vi "ParseIt.vi"(10 "Header Info":T1={"TFRFHeader"={"index"=22, "Xr"=294.1319931548027, "Yr"=349.0, "XActual"=294.1319931548027, "YActual"=349.0}, "Frequency Axis"={"Hz Resolution"=0.67291259765625, "Start Freq"=24.89776611328125, "End Freq"=3500.4913330078125}, "TSingleArray"={"fComplex"=1, "fLength"=5166.0, "a[2]"=0.0, "fConditionCheck"=1.0, "Precision"=0.0, "MtxVecVersion"=420.0, "SizeOf(TSample)"=8.0, "Tag"=0.0, "MtxVecFileCode"=64019.0, "a[9]"=0.0, "a[10]"=0.0}, "caption"="\u0000\u0000\u0000\u0000"}, 11 "Array":dbl[](array[numeric])) -> (1 "Waveform Graph":T2(graph), 2 "coherence":T2(graph), 3 "output array":dbl[][](array[numeric]), 4 "Complex FRF":cluster{"t0":dbl, "dt":dbl, "Y":cdb[]}, 5 "Number of bytes":dbl, 6 "run":cluster{"Sampling rate":dbl, "npts":dbl})   [LabVIEW 2022 SP3]
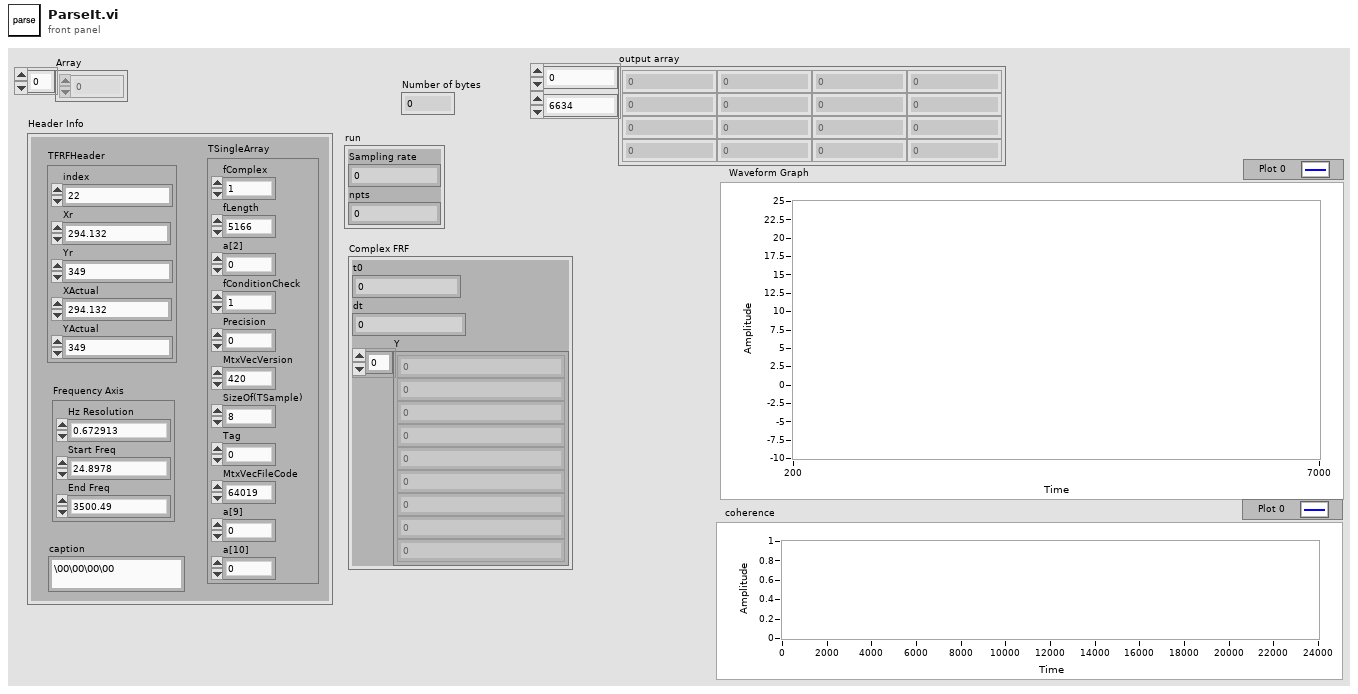
[diagram p1: front panel]
types:
  T1 = cluster{"TFRFHeader":cluster{"index":u32, "Xr":dbl, "Yr":dbl, "XActual":dbl, "YActual":dbl}, "Frequency Axis":cluster{"Hz Resolution":dbl, "Start Freq":dbl, "End Freq":dbl}, "TSingleArray":cluster{"fComplex":u32, "fLength":dbl, "a[2]":dbl, "fConditionCheck":dbl, "Precision":dbl, "MtxVecVersion":dbl, "SizeOf(TSample)":dbl, "Tag":dbl, "MtxVecFileCode":dbl, "a[9]":dbl, "a[10]":dbl}, "caption":string}
  T2 = cluster{"Start freq":dbl, "Hz resolution":dbl, dbl[]}
  T3 = cluster{"Start Freq":dbl, "Hz Resolution":dbl, cdb[]}
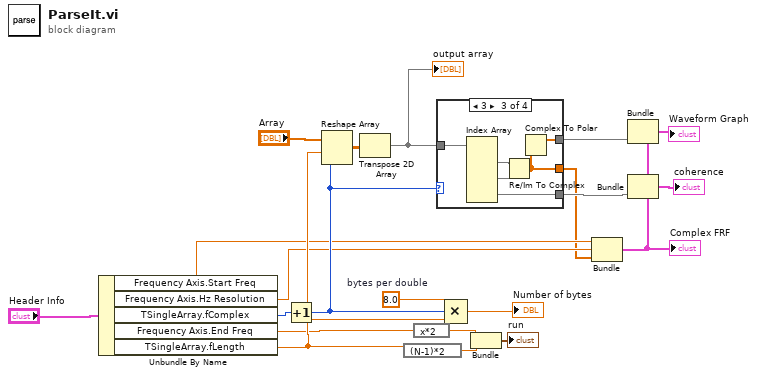
[diagram p0: block diagram]
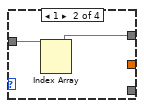
[diagram p3: hidden frame]
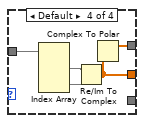
[diagram p4: hidden frame]
diagram:
  w11 = 8.0  # bytes per double
  n1 = Unbundle By Name("Header Info") -> ("Frequency Axis.Start Freq"=w3:dbl, "Frequency Axis.Hz Resolution"=w4:dbl, "TSingleArray.fComplex"=w16:u32, "Frequency Axis.End Freq"=w9:dbl, "TSingleArray.fLength"=w17:dbl)
  n2 = Increment(x=w16) -> (x+1=w19:u32)
  n3 = Reshape Array("Array", w17, w19) -> (w18:dbl[][])
  n4 = Transpose 2D Array(2D array=w18) -> (transposed array=w20:dbl[][])
  "output array" <- w20
  n5 = expression code="(N-1)*2"(w17) -> (w10:dbl)
  n6 = expression code="x*2"(w9) -> (w7:dbl)
  n7 = case shown="3" w19 {
    tunnel: w20 -> [_ w23 w29 w34]
    tunnel: [_ w22 w26 w31] -> w1
    tunnel: [_ _ w25 _] -> w21
    tunnel: [_ _ w24 w30] -> w2
    frame 0 {
    }
    frame 1 {
      n8 = Index Array(array=w23) -> (element=w22:dbl[])  [unwired: 2 in]
    }
    frame 3 {
      n9 = Index Array(array=w29) -> (element #1=w28:dbl[], element #2=w27:dbl[], element #3=w25:dbl[])  [unwired: 6 in]
      n10 = Re/Im To Complex(1:w27, 2:w28) -> (0:w24:cdb[])
      n11 = Complex To Polar(r * e^(i*theta)=w24) -> (r=w26:dbl[])  [unwired: 1 out]
    }
    frame Default {
      n12 = Index Array(array=w34) -> (element #1=w33:dbl[], element #2=w32:dbl[])  [unwired: 4 in]
      n13 = Re/Im To Complex(1:w32, 2:w33) -> (0:w30:cdb[])
      n14 = Complex To Polar(r * e^(i*theta)=w30) -> (r=w31:dbl[])  [unwired: 1 out]
    }
  }
  n15 = Compound Arithmetic op=MULTIPLY(w11, w19, w17) -> (→"Number of bytes":dbl)
  n16 = Bundle("End Freq"=w7, "fLength"=w10) -> (→"run":cluster{"End Freq":dbl, "fLength":dbl})  [unwired: 1 in]
  n17 = Bundle("Start Freq"=w3, "Hz Resolution"=w4, w2) -> (w12:T3)  [unwired: 1 in]
  "Complex FRF" <- w12
  n18 = Bundle(cluster=w12, w1) -> (→"Waveform Graph":T3)  [unwired: 2 in]
  n19 = Bundle(cluster=w12, w21) -> (→"coherence":T3)  [unwired: 2 in]
